vi "Send.vi"(8 "error in (no error)":errorcluster, 10 "Message":refnum<class "MSG.lvclass">, 11 "CancelableObserver":refnum<class "CancelableObserver.lvclass">) -> (0 "error out":errorcluster, 3 "CancelableObserver":refnum<class "CancelableObserver.lvclass">)   [LabVIEW 2011, in "Messenging.lvlib" / "CancelableObserver.lvclass"]
uses:
  CancelableObserver.lvclass
  SendOnly/Observer.lvclass
  TextVarientMessage/MSG.lvclass
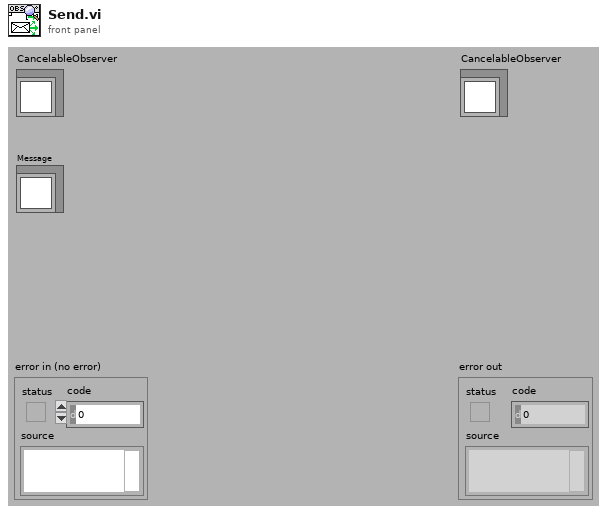
[diagram p1: front panel]
types:
  T1 = typedef "Semaphore RefNum" = refnum<k1>
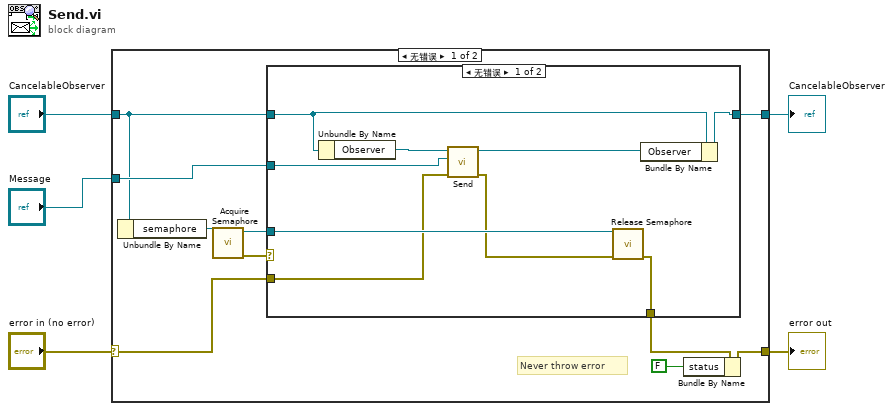
[diagram p0: block diagram]
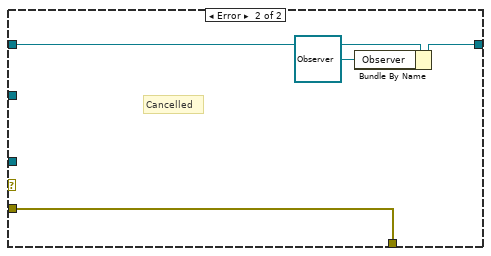
[diagram p2: hidden frame]
diagram:
  n1 = case shown="无错误" "error in (no error)" {
    selector: "error in (no error)" -> [w8 w29]
    tunnel: [w15 w30] -> w5
    tunnel: "Message" -> [w14 _]
    tunnel: "CancelableObserver" -> [w13 w30]
    tunnel: [w7 w29] -> w1
    frame No Error {
      # "Never throw error"
      n2 = Unbundle By Name(w13) -> ("semaphore"=w12:T1)
      n3 = call <vilib>:"Acquire Semaphore.vi"("semaphore"=w12) -> ("error out"=w11:errorcluster, "semaphore out"=w10:T1)  [unwired: 2 in, 3 out]
      n4 = case shown="无错误" w11 {
        tunnel: [w23 w27] -> w15
        tunnel: w14 -> [w19 _]
        tunnel: w13 -> [w22 w28]
        tunnel: w10 -> [w24 _]
        tunnel: [w17 w25] -> w9
        tunnel: w8 -> [w16 w25]
        frame No Error {
          n5 = Unbundle By Name(w22) -> ("Observer"=w21:refnum<class "Observer.lvclass">)
          n6 = call-dynamic "Send.vi"("error in (no error)"=w16, "Message"=w19, "MSR Parent in"=w21) -> ("error out"=w18:errorcluster, "MSR Parent out"=w20:refnum<class "Observer.lvclass">)  [unwired: 7 out]
          n7 = call <vilib>:"Release Semaphore.vi"("error in (no error)"=w18, "semaphore"=w24) -> ("error out"=w17:errorcluster)  [unwired: 5 out]
          n8 = Bundle By Name(cluster=w22, "Observer"=w20) -> (w23:refnum<class "CancelableObserver.lvclass">)
        }
        frame Error {
          # "Cancelled"
          n9 = Bundle By Name(cluster=w28, "Observer"=refnum<class "Observer.lvclass"> refnum ("ObserverSet")) -> (w27:refnum<class "CancelableObserver.lvclass">)
        }
      }
      n10 = Bundle By Name(cluster=w9, "status"=FALSE) -> (w7:errorcluster)
    }
    frame Error {
    }
  }
  "error out" <- w1
  "CancelableObserver" <- w5
